vi "getSoundPath.vi"(8 "error in (no error)":errorcluster, 11 "FileNeologist in":refnum<class "FileNeologist.lvclass">) -> (0 "error out":errorcluster, 2 "Path":path, 3 "FileNeologist out":refnum<class "FileNeologist.lvclass">)   [LabVIEW 2009, in "Tools.lvlib" / "Filing.lvlib" / "FileNeologist.lvclass"]
uses:
  FileNeologist.lvclass
  FileNeologist.lvclass/FileNeologist.ctl
  FileSystem/FileSystem.lvclass
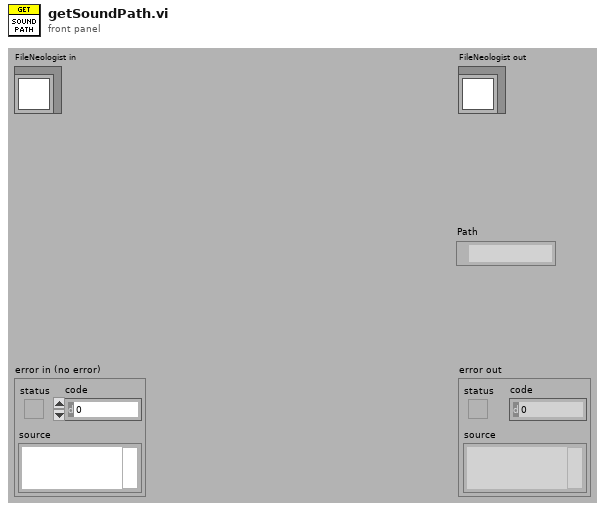
[diagram p1: front panel]
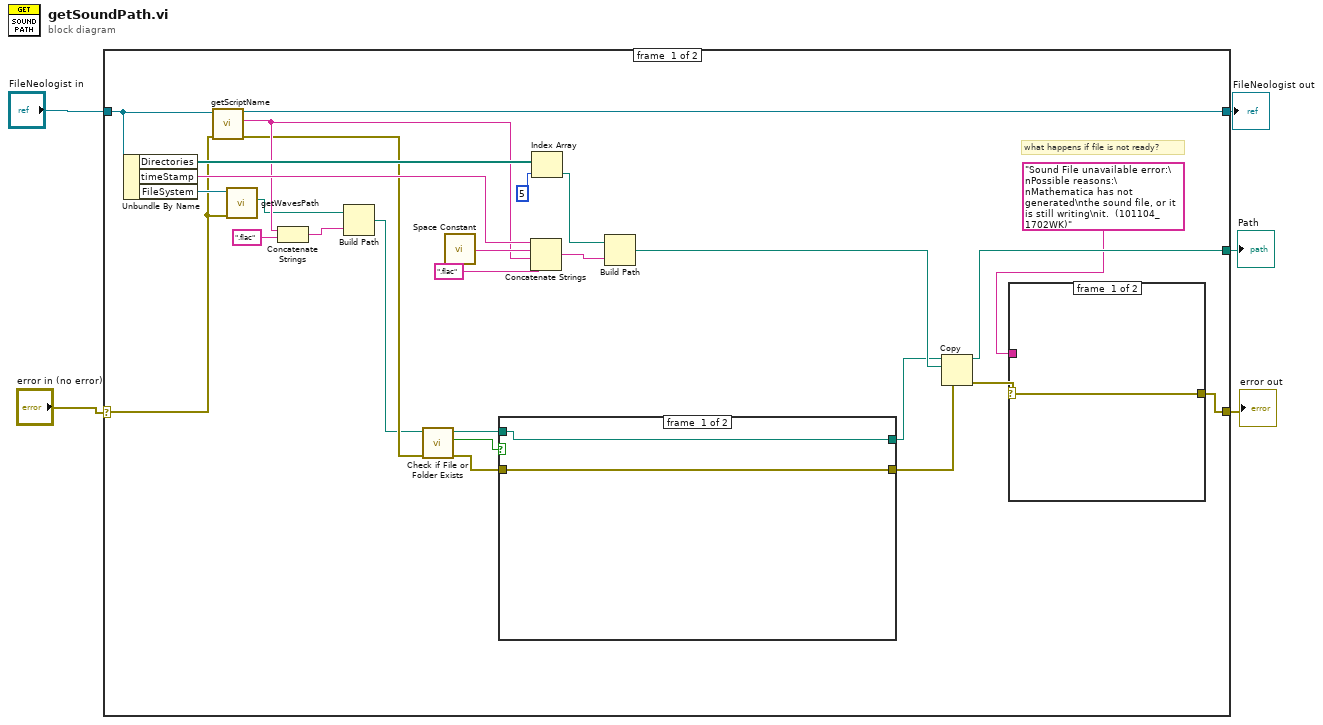
[diagram p0: block diagram]
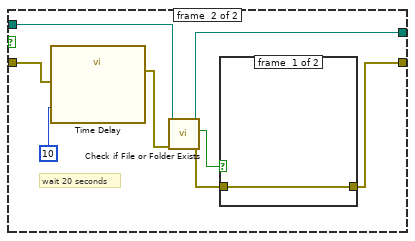
[diagram p2: hidden frame]
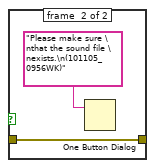
[diagram p3: hidden frame]
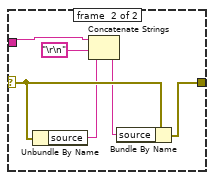
[diagram p4: hidden frame]
diagram:
  n1 = case shown="No Error" "error in (no error)" {
    selector: "error in (no error)" -> [w22 w54]
    tunnel: [w14 w54] -> w4
    tunnel: [w27 w53] -> w2
    tunnel: "FileNeologist in" -> [w28 w53]
    tunnel: [w16 _] -> w1
    frame #0 {
      # "what happens if file is not ready?"
      n2 = Unbundle By Name(w28) -> ("Directories"=w29:path[], "timeStamp"=w31:string, "FileSystem"=w23:refnum<class "FileSystem.lvclass">)
      n3 = call-dynamic "getScriptName.vi"("error in (no error)"=w22, "FileNeologist.lvclass in"=w28) -> ("error out"=w10:errorcluster, "scriptName"=w21:string, "FileNeologist.lvclass out"=w27:refnum<class "FileNeologist.lvclass">)  [unwired: 7 in]
      n4 = call "getWavesPath.vi"("error in (no error)"=w22, "FileSystem.lvclass in"=w23) -> ("Waves"=w19:path)  [unwired: 7 in, 2 out]
      n5 = Concatenate Strings(w21, ".flac") -> (w18:string)
      n6 = Build Path(base path=w19, name or relative path=w18) -> (appended path=w9:path)
      n7 = call <vilib>:"Check if File or Folder Exists.vi"("error in (no error)"=w10, "path"=w9) -> ("error out"=w11:errorcluster, "file or folder exists?"=w12:bool, "dup path"=w7:path)  [unwired: 7 in]
      n8 = call <vilib>:"Space Constant.vi"() -> ("String"=w32:string)
      n9 = case shown="False" w12 {
        tunnel: w11 -> [w34 w42]
        tunnel: [w34 w39] -> w8
        tunnel: w7 -> [w33 w38]
        tunnel: [w33 w37] -> w6
        frame #0 {
        }
        frame #1 {
          # "wait 20 seconds"
          n10 = call "Time Delay"("error in (no error)"=w42, "Delay Time (s)"=10) -> ("error out"=w41:errorcluster)  [unwired: 9 in]
          n11 = call <vilib>:"Check if File or Folder Exists.vi"("error in (no error)"=w41, "path"=w38) -> ("error out"=w40:errorcluster, "file or folder exists?"=w36:bool, "dup path"=w37:path)  [unwired: 7 in]
          n12 = case shown="False" w36 {
            tunnel: w40 -> [w43 w44]
            tunnel: [w43 w44] -> w39
            frame #0 {
            }
            frame #1 {
              n13 = One Button Dialog(message="Please make sure \nthat the sound file \nexists.\n(101105_0956WK)") -> ()  [unwired: 1 in, 1 out]
            }
          }
        }
      }
      n14 = Concatenate Strings(w31, w32, w21, ".flac") -> (w30:string)
      n15 = Index Array(array=w29, index=5) -> (element=w24:path)
      n16 = Build Path(base path=w24, name or relative path=w30) -> (appended path=w17:path)
      n17 = Copy(8:w8, 10:w17, 11:w6) -> (0:w15:errorcluster, 3:w16:path)  [unwired: 2 in, 1 out]
      n18 = case shown="Error" w15 {
        selector: w15 -> [w46 w52]
        tunnel: [w46 w51] -> w14
        tunnel: "Sound File unavailable error:\nPossible reasons:\nMathematica has not generated\nthe sound file, or it is still writing\nit.  (101104_1702WK)" -> [_ w47]
        frame #0 {
        }
        frame #1 {
          n19 = Unbundle By Name(w52) -> ("source"=w50:string)
          n20 = Concatenate Strings(w47, "\r\n", w50) -> (w49:string)
          n21 = Bundle By Name(cluster=w52, "source"=w49) -> (w51:errorcluster)
        }
      }
    }
    frame #1 {
    }
  }
  "error out" <- w4
  "FileNeologist out" <- w2
  "Path" <- w1
